vi "Configure Power Analysis (Efficiency).vi"(8 "error in (no error)":errorcluster, 10 "Power Efficiency Type (0: DCDC)":i32(ring) items=["DCDC", "DCAC", "ACDC", "ACAC"], 11 "VISA resource name":refnum<visa-resource-name>) -> (0 "error out":errorcluster, 3 "VISA resource name out":refnum<visa-resource-name>)   [LabVIEW 2023, in "Keysight-DSQx3014T.lvlib"]
doc: "Applies the effieciency power analysis.\n\n<B>Note(s):</B>\nEfficiency analysis tests the overall efficiency of the power supply by measuring the output power over the input power.\n\nUse <B>Read Measurement (Efficiency Power Analysis).vi</B> to read the result of this power analysis."
uses:
  Keysight-DSQx3014T.lvlib
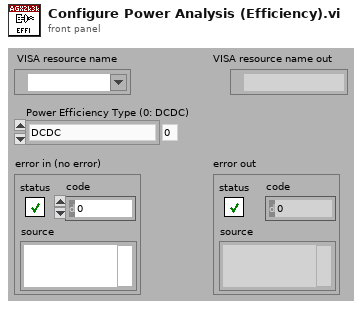
[diagram p1: front panel]
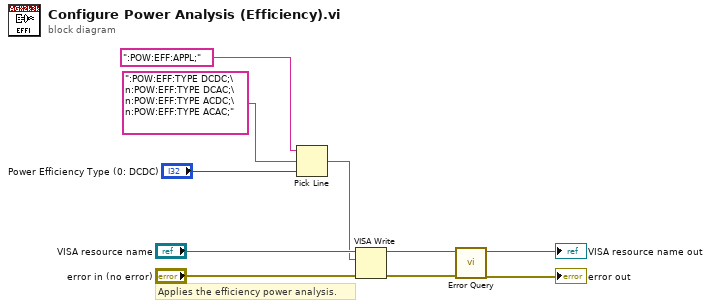
[diagram p0: block diagram]
diagram:
  # "Applies the efficiency power analysis."
  n1 = Pick Line(string ("")=":POW:EFF:APPL;", multi-line string=":POW:EFF:TYPE DCDC;\n:POW:EFF:TYPE DCAC;\n:POW:EFF:TYPE ACDC;\n:POW:EFF:TYPE ACAC;", line index="Power Efficiency Type (0: DCDC)") -> (output string=w1:string)
  n2 = VISA Write(VISA resource name="VISA resource name", write buffer=w1, error in (no error)="error in (no error)") -> (VISA resource name out=w8:refnum<visa-resource-name>, error out=w7:errorcluster)  [unwired: 1 out]
  n3 = call "Error Query.vi"("error in (no error)"=w7, "VISA resource name"=w8) -> ("error out"=→"error out":errorcluster, "VISA resource name out"=→"VISA resource name out":refnum<visa-resource-name>)  [unwired: 8 out]
